vi "Read Meta Data.vi"(8 "error in (no error)":errorcluster, 11 "Message in":refnum<class "Message.lvclass">) -> (0 "error out":errorcluster, 1 "Sender":string, 2 "Time Stamp":timestamp, 3 "Message out":refnum<class "Message.lvclass">)   [LabVIEW 2015, in "Message.lvclass"]
uses:
  Message.lvclass
  Message.lvclass/Message.ctl
panel:
  out "Sequence Number":u64
  out "Name":string
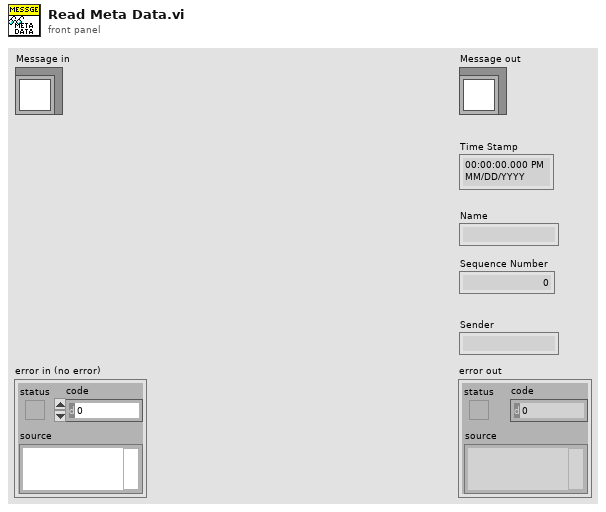
[diagram p1: front panel]
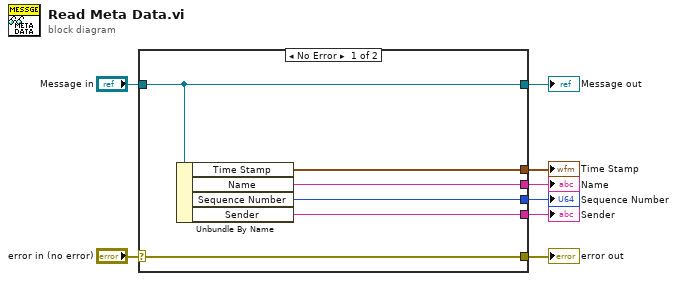
[diagram p0: block diagram]
diagram:
  n1 = case shown="No Error" "error in (no error)" {
    selector: "error in (no error)" -> [w14 w15]
    tunnel: [w14 w15] -> w7
    tunnel: [w13 w16] -> w5
    tunnel: "Message in" -> [w13 w16]
    tunnel: [w12 _] -> w4
    tunnel: [w11 _] -> w3
    tunnel: [w10 _] -> w2
    tunnel: [w9 _] -> w1
    frame No Error {
      n2 = Unbundle By Name(w13) -> ("Time Stamp"=w12:timestamp, "Name"=w11:string, "Sequence Number"=w10:u64, "Sender"=w9:string)
    }
    frame Error {
    }
  }
  "error out" <- w7
  "Message out" <- w5
  "Time Stamp" <- w4
  "Name" <- w3
  "Sequence Number" <- w2
  "Sender" <- w1
